vi "create.vi"(8 "error in (no error)":errorcluster, 11 "Type":T1=enum."PSU_NI") -> (0 "error out":errorcluster, 3 "PowerSupply.lvclass":refnum<class "PowerSupply.lvclass">)   [LabVIEW 2023, in "swePsu.lvlib"]
doc: "Create a new powersupply object."
uses:
  swePsu.lvlib
  Data/PsuTypes.ctl
  PowerSupply.lvclass
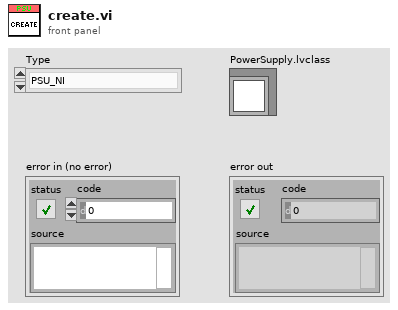
[diagram p1: front panel]
types:
  T1 = typedef "swePsu.lvlib/PsuTypes.ctl" = enum16{"Simulated", "PSU_NI", "PSU_TTi"}
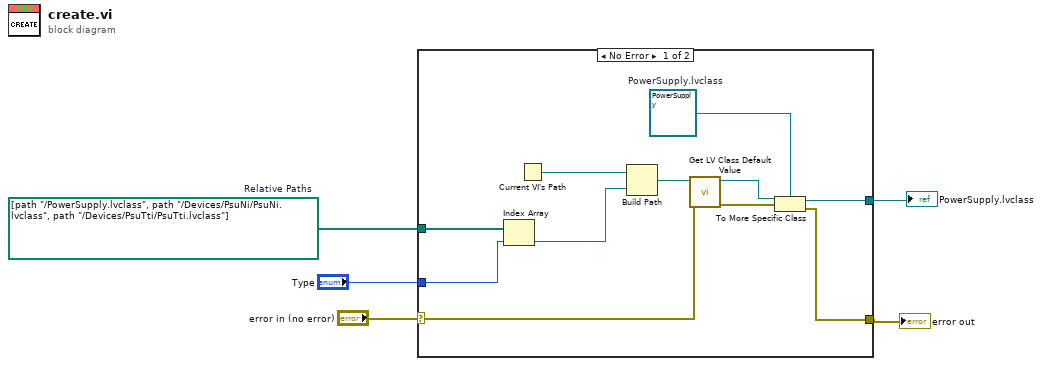
[diagram p0: block diagram]
diagram:
  w1 = path[] [path "../PowerSupply.lvclass", path "../Devices/PsuNi/PsuNi.lvclass", path "../Devices/PsuTti/PsuTti.lvclass"]  # Relative Paths
  n1 = case shown="No Error" "error in (no error)" {
    selector: "error in (no error)" -> [w15 w17]
    tunnel: [w13 _] -> w5
    tunnel: w1 -> [w12 _]
    tunnel: "Type" -> [w10 _]
    tunnel: [w7 w17] -> w4
    frame No Error {
      w6 = refnum<class "PowerSupply.lvclass"> refnum  # PowerSupply.lvclass
      n2 = Index Array "Index Array"(array=w12, index=w10) -> (element=w11:path)
      n3 = Current VI's Path() -> (path=w16:path)
      n4 = Build Path(base path=w16, name or relative path=w11) -> (appended path=w14:path)
      n5 = call <vilib>:"Get LV Class Default Value.vi"("error in (no error)"=w15, "class path"=w14) -> ("error out"=w9:errorcluster, "object"=w8:refnum<class>)  [unwired: 8 in]
      n6 = To More Specific Class(target class=w6, reference=w8, error in=w9) -> (specific class reference=w13:refnum<class "PowerSupply.lvclass">, error out=w7:errorcluster)
    }
    frame Error {
    }
  }
  "error out" <- w4
  "PowerSupply.lvclass" <- w5
